vi "PollReceiveQueue.vi"(8 "error in (no error)":errorcluster, 9 "keep semaphore":bool, 10 "waiting time ms (-1: forever)":i32=10, 11 "queue cluster":T1) -> (0 "semaphore error out":errorcluster, 1 "receive queue error out":errorcluster, 2 "# elements in queue":i32, 3 "receive queue":refnum<queue>)   [LabVIEW 2014]
uses:
  typedefs/QueueCluster.ctl
  typedefs/clientStatus.ctl
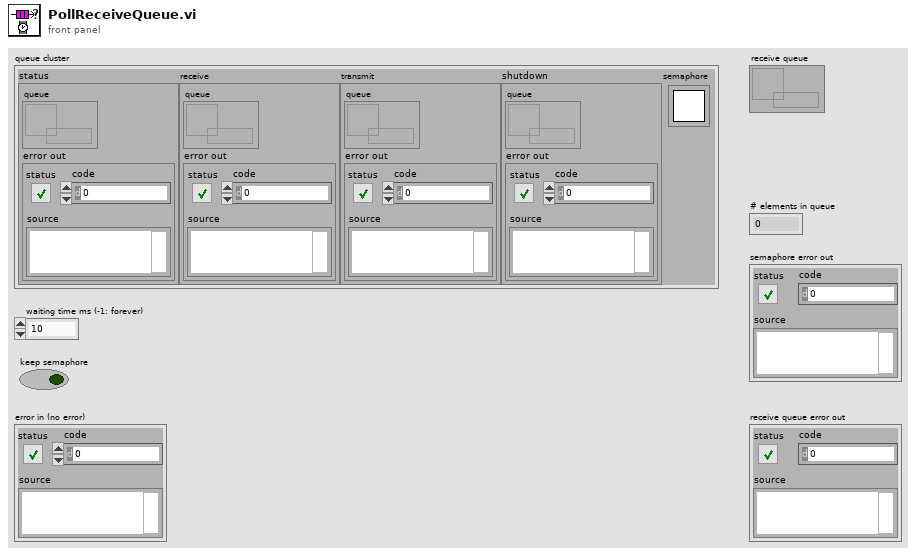
[diagram p1: front panel]
types:
  T1 = typedef "QueueCluster.ctl" = cluster{"status":cluster{"queue":refnum<queue>, "error out":errorcluster}, "receive":cluster{"queue":refnum<queue>, "error out":errorcluster}, "transmit":cluster{"queue":refnum<queue>, "error out":errorcluster}, "shutdown":cluster{"queue":refnum<queue>, "error out":errorcluster}, "semaphore":T2}
  T2 = typedef "Semaphore RefNum" = refnum<k1>
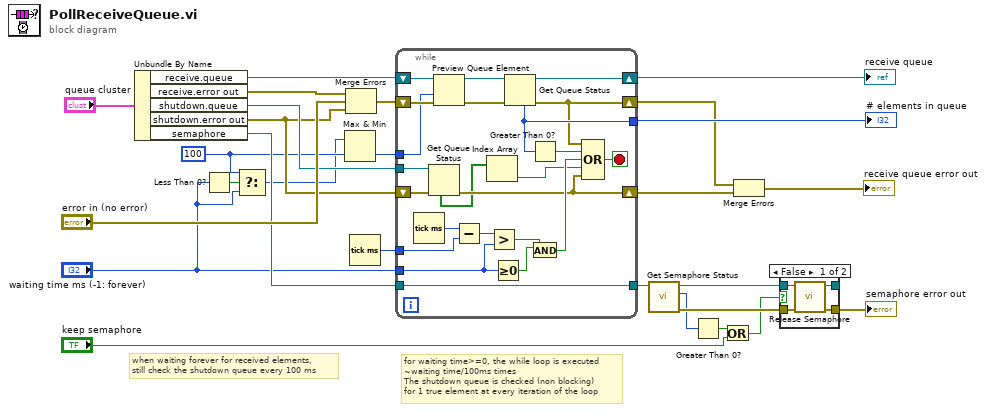
[diagram p0: block diagram]
diagram:
  w2 = 100 ("t")
  # "when waiting forever for received elements,\nstill check the shutdown queue every 100 ms"
  # "for waiting time>=0, the while loop is executed\n~waiting time/100ms times\nThe shutdown queue is checked (non blocking)\nfor 1 true element at every iteration of the loop"
  n1 = Unbundle By Name("queue cluster") -> ("receive.queue"=w13:refnum<queue>, "receive.error out"=w16:errorcluster, "shutdown.queue"=w11:refnum<queue>, "shutdown.error out"=w6:errorcluster, "semaphore"=w10:T2)
  n2 = Less Than 0?(x="waiting time ms (-1: forever)") -> (x < 0?=w5:bool)
  n3 = Select(t=w2, s=w5, f="waiting time ms (-1: forever)") -> (s? t:f=w1:i32)
  n4 = Max & Min(x=w1, y=w2) -> (min(x,y)=w3:i32)  [unwired: 1 out]
  n5 = Merge Errors(w16, "error in (no error)", w6) -> (w15:errorcluster)
  n6 = Tick Count (ms)() -> (millisecond timer value=w18:u32)
  n7 = while {
    tunnel: [w48] -> w19
    shift-right: [w50] -> w14
    shift-left: w13 -> [w37]
    shift-right: [w42] -> w8
    shift-left: w15 -> [w36]
    tunnel: w18 -> [w46]
    tunnel: "waiting time ms (-1: forever)" -> [w41]
    tunnel: [w43] -> w27
    tunnel: w10 -> [w43]
    tunnel: w11 -> [w32]
    shift-right: [w30] -> w9
    shift-left: w6 -> [w31]
    tunnel: w3 -> [w33]
    stop <- w44 stop-if-true
    n8 = Tick Count (ms)() -> (millisecond timer value=w47:u32)
    n9 = Get Queue Status(queue=w32, error in (no error)=w31) -> (error out=w30:errorcluster, elements=w28:bool[])  [unwired: 1 in, 6 out]
    n10 = Preview Queue Element(queue=w37, timeout in ms (-1)=w33, error in (no error)=w36) -> (queue out=w35:refnum<queue>, error out=w34:errorcluster)  [unwired: 2 out]
    n11 = Subtract(x=w47, y=w46) -> (x-y=w45:u32)
    n12 = Index Array(array=w28) -> (element=w29:bool)  [unwired: 1 in]
    n13 = Greater?(x=w45, y=w41) -> (0:w39:bool)
    n14 = Greater Or Equal To 0?(x=w41) -> (x >= 0?=w40:bool)
    n15 = Get Queue Status(queue=w35, error in (no error)=w34) -> (queue out=w50:refnum<queue>, error out=w42:errorcluster, # elements in queue=w48:i32)  [unwired: 1 in, 5 out]
    n16 = Greater Than 0?(x=w48) -> (x > 0?=w49:bool)
    n17 = And(x=w39, y=w40) -> (x .and. y?=w38:bool)
    n18 = Compound Arithmetic op=OR(w42, w49, w38, w29, w30) -> (w44:bool)
  }
  "# elements in queue" <- w19
  "receive queue" <- w14
  n19 = call <vilib>:"Get Semaphore Status.vi"("semaphore"=w27) -> ("error out"=w25:errorcluster, "# available"=w20:i32, "semaphore out"=w22:T2)  [unwired: 5 in, 3 out]
  n20 = Greater Than 0?(x=w20) -> (x > 0?=w21:bool)
  n21 = Or(x=w21, y="keep semaphore") -> (x .or. y?=w24:bool)
  n22 = Merge Errors(w8, w9) -> (→"receive queue error out":errorcluster)
  n23 = case shown="False" w24 {
    tunnel: w22 -> [w54 w56]
    tunnel: [w53 w56] -> _
    tunnel: w25 -> [w52 w55]
    tunnel: [w51 w55] -> w26
    frame False {
      n24 = call <vilib>:"Release Semaphore.vi"("error in (no error)"=w52, "semaphore"=w54) -> ("error out"=w51:errorcluster, "semaphore out"=w53:T2)  [unwired: 4 in]
    }
    frame True {
    }
  }
  "semaphore error out" <- w26
